vi "LDT Parse XML Status.vi"(8 "error in":errorcluster, 11 "XML Status":string="<tcsTCSStatus>\n  <tcsVersion>V1.8</tcsVersion>\n  <accessMode>Operator</accessMode>\n  <azCurrentWrap>-1</azCurrentWrap>\n  <heartbeat>2081334</heartbeat>\n  <inPositionIsTrue>true</inPositionIsTrue>\n  <m1CoverState>Closed</m1CoverState>\n  <mountGuideMode>OpenLoop</mountGuideMode>\n  <rotCurrentWrap>-1</rotCurrentWrap>\n  <tcsHealth>WARNING</tcsHealth>\n  <tcsState>ENABLED</tcsState>\n  <currentTimes>\n    <lst>\n      <hours>12</hours>\n      <minutesTime>55</minutesTime>\n      <secondsTime>41</secondsTime>\n    </lst>\n    <time>2020-09-14T20:44:15.228+00:00</time>\n  </currentTimes>\n  <limits>\n    <moonProximity>\n      <distance_deg>51.647106572866</distance_deg>\n      <proximityFlag>false</proximityFlag>\n    </moonProximity>\n    <sunProximity>\n      <distance_deg>16.531164188648</distance_deg>\n      <proximityFlag>false</proximityFlag>\n    </sunProximity>\n    <zenith>\n      <currentZD_deg>46.221286</currentZD_deg>\n      <elZenithLimit_deg>89.3</elZenithLimit_deg>\n      <inBlindSpotIsTrue>false</inBlindSpotIsTrue>\n      <timeToBlindSpot_min>-1</timeToBlindSpot_min>\n      <timeToBlindSpotExit_min>-1</timeToBlindSpotExit_min>\n    </zenith>\n    <airmass>1.4438282807451</airmass>\n    <currentTimeToObservable_min>-1</currentTimeToObservable_min>\n    <currentTimeToUnobservable_min>262</currentTimeToUnobservable_min>\n    <timeToRotLimit_min>-1</timeToRotLimit_min>\n    <timeToAzLimit_min>-1</timeToAzLimit_min>\n  </limits>\n  <pointingPositions>\n    <azElError>\n      <azError>-0.9792</azError>\n      <elError>0.1584</elError>\n    </azElError>\n    <currentAzEl>\n      <azimuth>\n        <degreesArc>194</degreesArc>\n        <minutesArc>45</minutesArc>\n        <secondsArc>0.7</secondsArc>\n      </azimuth>\n      <elevation>\n        <degreesAlt>43</degreesAlt>\n        <minutesArc>46</minutesArc>\n        <secondsArc>43.4</secondsArc>\n      </elevation>\n    </currentAzEl>\n    <currentHA>\n      <hours>0</hours>\n      <minutesTime>44</minutesTime>\n      <secondsTime>2.04</secondsTime>\n    </currentHA>\n    <currentRADec>\n      <declination>\n        <degreesDec>-10</degreesDec>\n        <minutesArc>15</minutesArc>\n        <secondsArc>25</secondsArc>\n      </declination>\n      <equinoxPrefix>J</equinoxPrefix>\n      <equinoxYear>2000</equinoxYear>\n      <frame>FK5</frame>\n      <ra>\n        <hours>12</hours>\n        <minutesTime>10</minutesTime>\n        <secondsTime>35.34</secondsTime>\n      </ra>\n    </currentRADec>\n    <currentParAngle>12.557342470137</currentParAngle>\n    <currentRotatorPositions>\n      <rotPA>342.260103</rotPA>\n      <iaa>185.2</iaa>\n      <rotIPA>0</rotIPA>\n    </currentRotatorPositions>\n    <difftrackStatus>\n      <dAz_ArcsPS>0</dAz_ArcsPS>\n      <dEl_ArcsPS>0</dEl_ArcsPS>\n      <dRA_ArcsPS>0</dRA_ArcsPS>\n      <dDec_ArcsPS>0</dDec_ArcsPS>\n    </difftrackStatus>\n    <objectPA>\n      <EqPA>-0</EqPA>\n      <AzPA>12.557342470137</AzPA>\n    </objectPA>\n    <demandAzEl>\n      <azimuth>\n        <degreesArc>194</degreesArc>\n        <minutesArc>45</minutesArc>\n        <secondsArc>3.68</secondsArc>\n      </azimuth>\n      <elevation>\n        <degreesAlt>43</degreesAlt>\n        <minutesArc>46</minutesArc>\n        <secondsArc>42.89</secondsArc>\n      </elevation>\n    </demandAzEl>\n    <demandRADec>\n      <declination>\n        <degreesDec>-10</degreesDec>\n        <minutesArc>15</minutesArc>\n        <secondsArc>25</secondsArc>\n      </declination>\n      <equinoxPrefix>J</equinoxPrefix>\n      <equinoxYear>2000</equinoxYear>\n      <frame>FK5</frame>\n      <ra>\n        <hours>12</hours>\n        <minutesTime>10</minutesTime>\n        <secondsTime>35.24</secondsTime>\n      </ra>\n    </demandRADec>\n    <demandRotatorPositions>\n      <rotPA>342.259442</rotPA>\n    </demandRotatorPositions>\n    <targetName>unspecified</targetName>\n  </pointingPositions>\n  <OffsetStatus>\n    <offsetType>SIMPLE</offsetType>\n    <userOff1>0</userOff1>\n    <userOff2>0</userOff2>\n    <handsetOff1>0</handsetOff1>\n    <handsetOff2>0</handsetOff2>\n  </OffsetStatus>\n  <axesTrackMode>All</axesTrackMode>\n  <inPositionAzIsTrue>true</inPositionAzIsTrue>\n  <inPositionElIsTrue>true</inPositionElIsTrue>\n  <inPositionRotIsTrue>true</inPositionRotIsTrue>\n  <externalTargetCfgCmdPreviewIsTrue>true</externalTargetCfgCmdPreviewIsTrue>\n</tcsTCSStatus>") -> (0 "error out":errorcluster, 3 "Telescope Status":T1)   [LabVIEW 2024, in "LDT Telescope.lvclass"]
uses:
  LDT Telescope.lvclass
  Telescope cluster Status.ctl
  typedefs/CC cluster RA and DEC.ctl
  Telescope enum Status.ctl
  Telescope.lvclass
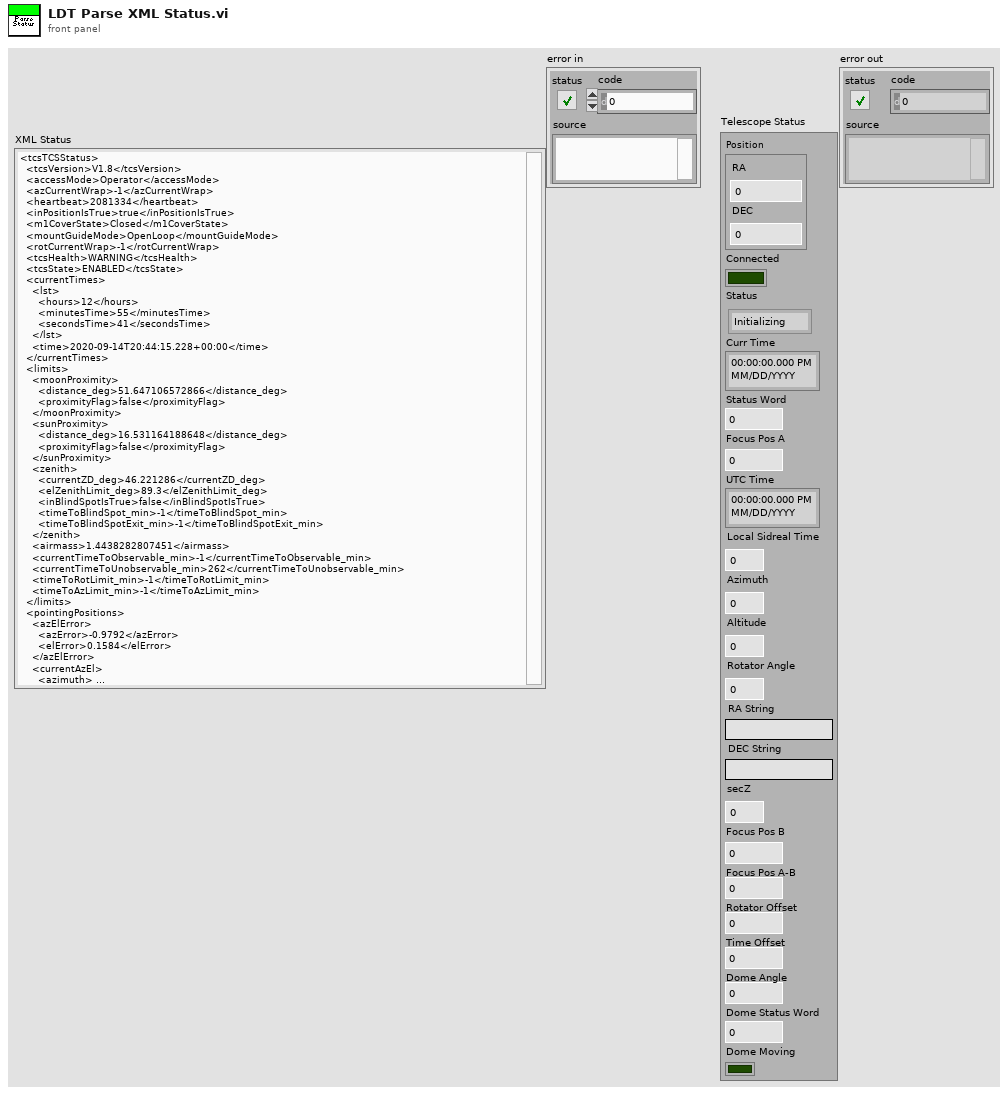
[diagram p1: front panel]
types:
  T1 = typedef "Telescope.lvclass/Telescope cluster Status.ctl" = cluster{"Position":T2, "Connected":bool, "Status":T3, "Curr Time":timestamp, "Status Word":u32, "Focus Pos A":dbl, "UTC Time":timestamp, "Local Sidreal Time":dbl, "Azimuth":dbl, "Altitude":dbl, "Rotator Angle":dbl, "RA String":string, "DEC String":string, "secZ":dbl, "Focus Pos B":dbl, "Focus Pos A-B":dbl, "Rotator Offset":dbl, "Time Offset":dbl, "Dome Angle":dbl, "Dome Status Word":u32, "Dome Moving":bool}
  T2 = typedef "CC cluster RA and DEC.ctl" = cluster{"RA":dbl, "DEC":dbl}
  T3 = typedef "Telescope.lvclass/Telescope enum Status.ctl" = enum16{"Initializing", "Ready", "Moving", "Focusing", "Error"}
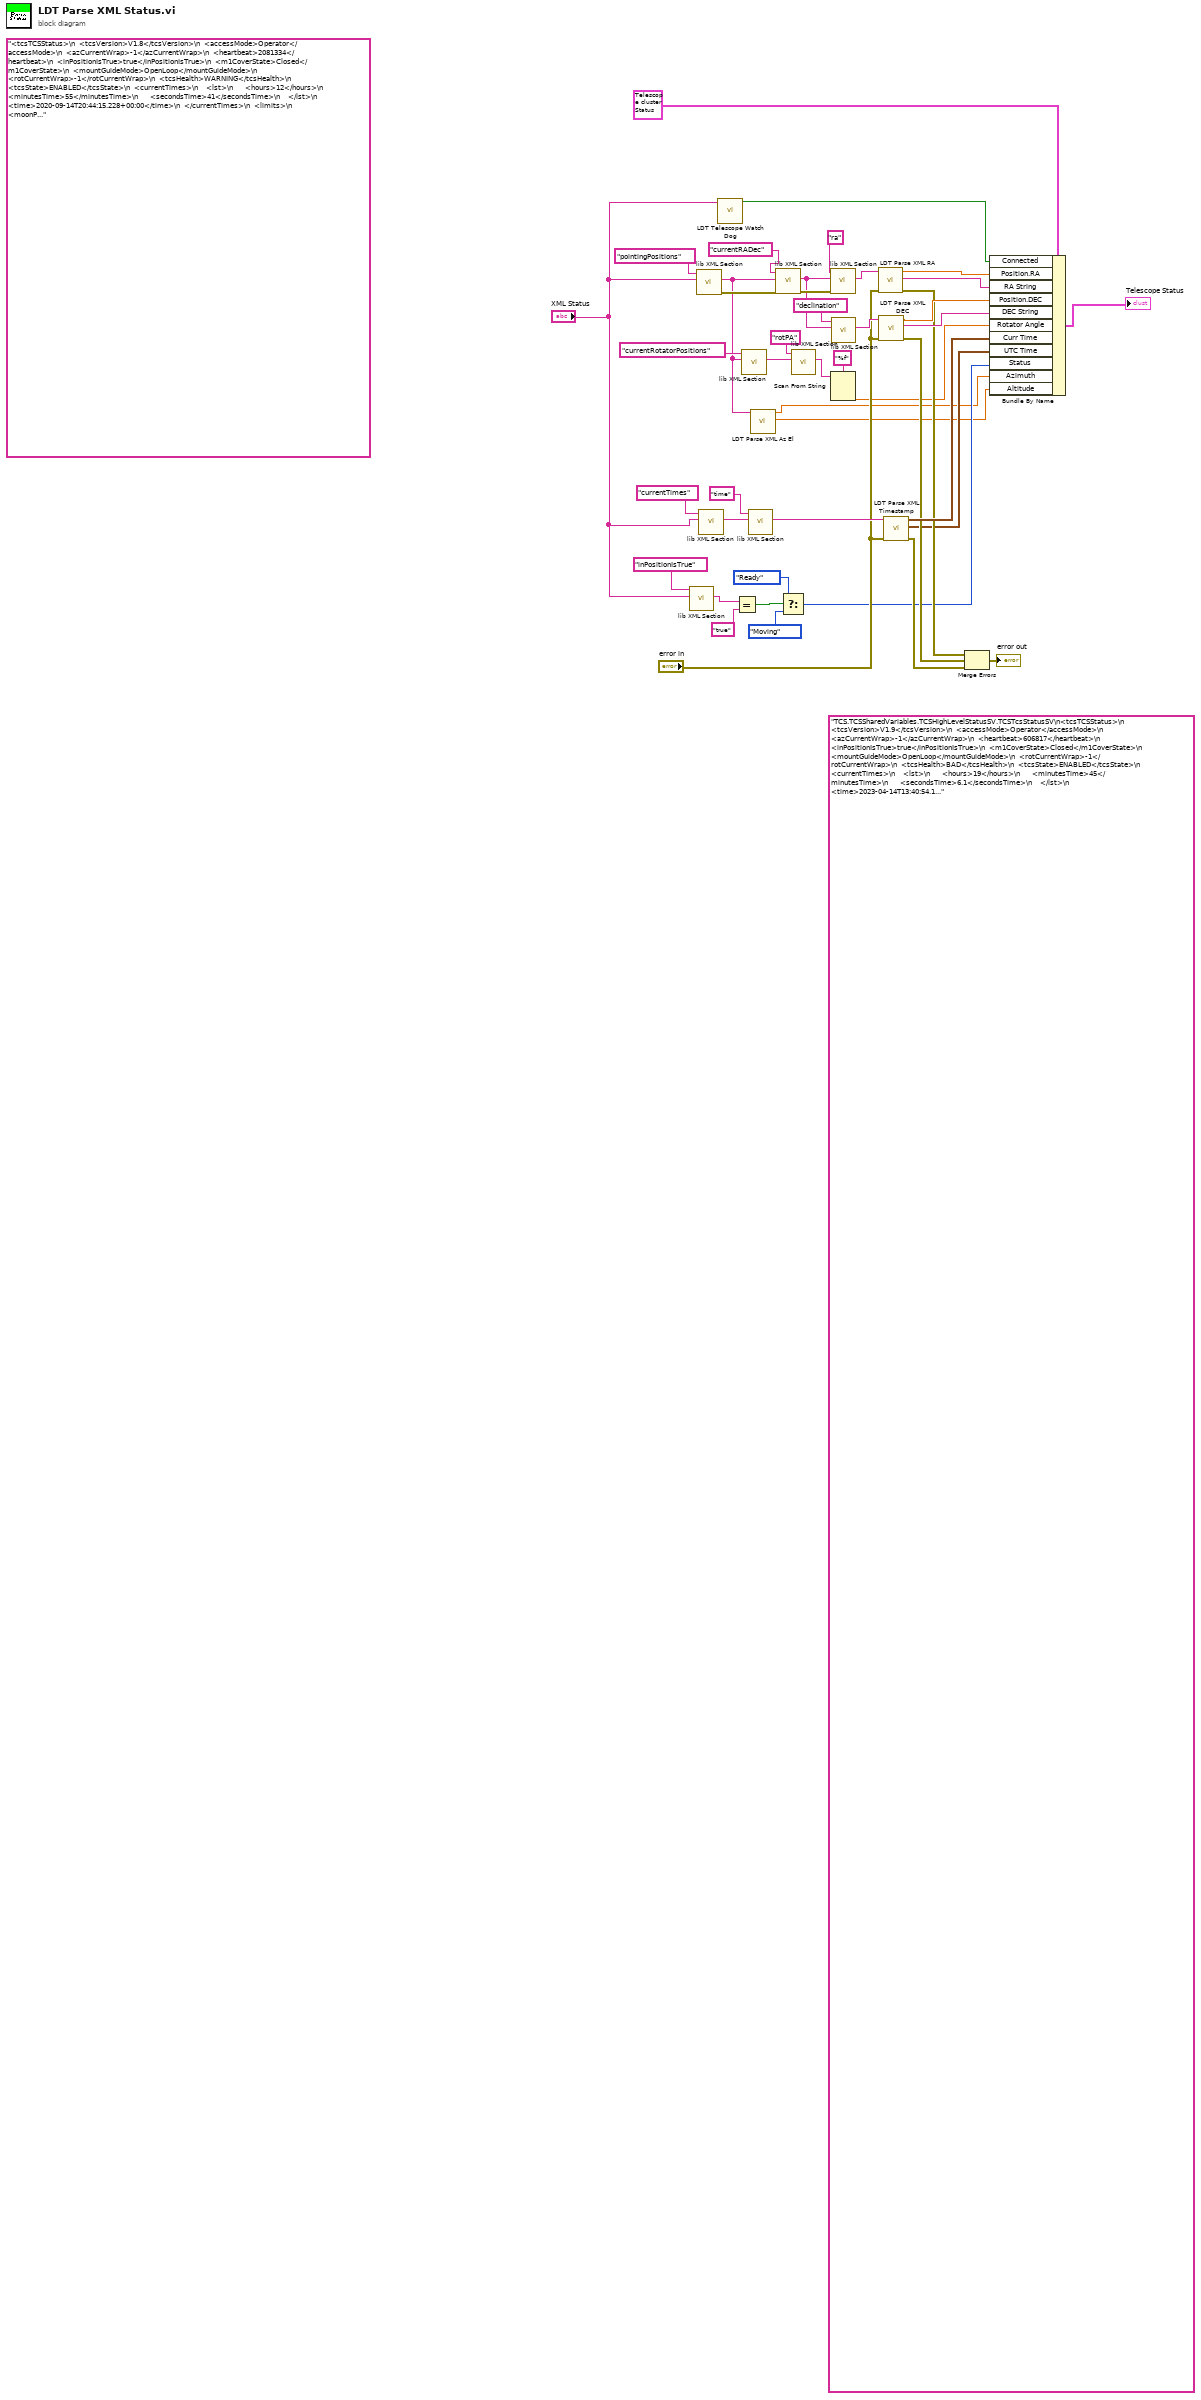
[diagram p0: block diagram]
diagram:
  (unwired) "TCS.TCSSharedVariables.TCSHighLevelStatusSV.TCSTcsStatusSV\n<tcsTCSStatus>\n  <tcsVersion>V1.9</tcsVersion>\n  <accessMode>Operator</accessMode>\n  <azCurrentWrap>-1</azCurrentWrap>\n  <heartbeat>606817</heartbeat>\n  <inPositionIsTrue>true</inPositionIsTrue>\n  <m1CoverState>Closed</m1CoverState>\n  <mountGuideMode>OpenLoop</mountGuideMode>\n  <rotCurrentWrap>-1</rotCurrentWrap>\n  <tcsHealth>BAD</tcsHealth>\n  <tcsState>ENABLED</tcsState>\n  <currentTimes>\n    <lst>\n      <hours>19</hours>\n      <minutesTime>45</minutesTime>\n      <secondsTime>6.1</secondsTime>\n    </lst>\n    <time>2023-04-14T13:40:54.171+00:00</time>\n  </currentTimes>\n  <limits>\n    <moonProximity>\n      <distance_deg>135.17188173454</distance_deg>\n      <proximityFlag>false</proximityFlag>\n    </moonProximity>\n    <sunProximity>\n      <distance_deg>85.698048093239</distance_deg>\n      <proximityFlag>false</proximityFlag>\n    </sunProximity>\n    <zenith>\n      <currentZD_deg>77.038641</currentZD_deg>\n      <elZenithLimit_deg>89.3</elZenithLimit_deg>\n      <inBlindSpotIsTrue>false</inBlindSpotIsTrue>\n      <timeToBlindSpot_min>-1</timeToBlindSpot_min>\n      <timeToBlindSpotExit_min>-1</timeToBlindSpotExit_min>\n    </zenith>\n    <airmass>4.3842110871255</airmass>\n    <currentTimeToObservable_min>-1</currentTimeToObservable_min>\n    <currentTimeToUnobservable_min>-1</currentTimeToUnobservable_min>\n    <timeToRotLimit_min>-1</timeToRotLimit_min>\n    <timeToAzLimit_min>-1</timeToAzLimit_min>\n  </limits>\n  <pointingPositions>\n    <azElError>\n      <azError>-0.288</azError>\n      <elError>0.036</elError>\n    </azElError>\n    <currentAzEl>\n      <azimuth>\n        <degreesArc>356</degreesArc>\n        <minutesArc>30</minutesArc>\n        <secondsArc>2.4</secondsArc>\n      </azimuth>\n      <elevation>\n        <degreesAlt>12</degreesAlt>\n        <minutesArc>57</minutesArc>\n        <secondsArc>40.9</secondsArc>\n      </elevation>\n    </currentAzEl>\n    <currentHA>\n      <hours>11</hours>\n      <minutesTime>26</minutesTime>\n      <secondsTime>48.74</secondsTime>\n    </currentHA>\n    <currentRADec>\n      <declination>\n        <degreesDec>68</degreesDec>\n        <minutesArc>0</minutesArc>\n        <secondsArc>0.3</secondsArc>\n      </declination>\n      <equinoxPrefix>J</equinoxPrefix>\n      <equinoxYear>2000</equinoxYear>\n      <frame>FK5</frame>\n      <ra>\n        <hours>8</hours>\n        <minutesTime>16</minutesTime>\n        <secondsTime>0.18</secondsTime>\n      </ra>\n    </currentRADec>\n    <currentParAngle>6.9879469176224</currentParAngle>\n    <currentRotatorPositions>\n      <rotPA>348.103896</rotPA>\n      <iaa>185.2</iaa>\n      <rotIPA>0</rotIPA>\n    </currentRotatorPositions>\n    <difftrackStatus>\n      <dAz_ArcsPS>0</dAz_ArcsPS>\n      <dEl_ArcsPS>0</dEl_ArcsPS>\n      <dRA_ArcsPS>0</dRA_ArcsPS>\n      <dDec_ArcsPS>0</dDec_ArcsPS>\n    </difftrackStatus>\n    <objectPA>\n      <EqPA>-0</EqPA>\n      <AzPA>6.9879469176224</AzPA>\n    </objectPA>\n    <demandAzEl>\n      <azimuth>\n        <degreesArc>356</degreesArc>\n        <minutesArc>30</minutesArc>\n        <secondsArc>3.57</secondsArc>\n      </azimuth>\n      <elevation>\n        <degreesAlt>12</degreesAlt>\n        <minutesArc>57</minutesArc>\n        <secondsArc>40.76</secondsArc>\n      </elevation>\n    </demandAzEl>\n    <demandRADec>\n      <declination>\n        <degreesDec>68</degreesDec>\n        <minutesArc>0</minutesArc>\n        <secondsArc>0.3</secondsArc>\n      </declination>\n      <equinoxPrefix>J</equinoxPrefix>\n      <equinoxYear>2000</equinoxYear>\n      <frame>FK5</frame>\n      <ra>\n        <hours>8</hours>\n        <minutesTime>16</minutesTime>\n        <secondsTime>0.03</secondsTime>\n      </ra>\n    </demandRADec>\n    <demandRotatorPositions>\n      <rotPA>348.104592</rotPA>\n    </demandRotatorPositions>\n    <targetName>MyTarget</targetName>\n  </pointingPositions>\n  <OffsetStatus>\n    <offsetType>SIMPLE</offsetType>\n    <userOff1>0</userOff1>\n    <userOff2>0</userOff2>\n    <handsetOff1>0</handsetOff1>\n    <handsetOff2>0</handsetOff2>\n  </OffsetStatus>\n  <axesTrackMode>All</axesTrackMode>\n  <inPositionAzIsTrue>true</inPositionAzIsTrue>\n  <inPositionElIsTrue>true</inPositionElIsTrue>\n  <inPositionRotIsTrue>true</inPositionRotIsTrue>\n  <externalTargetCfgCmdPreviewIsTrue>true</externalTargetCfgCmdPreviewIsTrue>\n</tcsTCSStatus>"
  (unwired) "<tcsTCSStatus>\n  <tcsVersion>V1.8</tcsVersion>\n  <accessMode>Operator</accessMode>\n  <azCurrentWrap>-1</azCurrentWrap>\n  <heartbeat>2081334</heartbeat>\n  <inPositionIsTrue>true</inPositionIsTrue>\n  <m1CoverState>Closed</m1CoverState>\n  <mountGuideMode>OpenLoop</mountGuideMode>\n  <rotCurrentWrap>-1</rotCurrentWrap>\n  <tcsHealth>WARNING</tcsHealth>\n  <tcsState>ENABLED</tcsState>\n  <currentTimes>\n    <lst>\n      <hours>12</hours>\n      <minutesTime>55</minutesTime>\n      <secondsTime>41</secondsTime>\n    </lst>\n    <time>2020-09-14T20:44:15.228+00:00</time>\n  </currentTimes>\n  <limits>\n    <moonProximity>\n      <distance_deg>51.647106572866</distance_deg>\n      <proximityFlag>false</proximityFlag>\n    </moonProximity>\n    <sunProximity>\n      <distance_deg>16.531164188648</distance_deg>\n      <proximityFlag>false</proximityFlag>\n    </sunProximity>\n    <zenith>\n      <currentZD_deg>46.221286</currentZD_deg>\n      <elZenithLimit_deg>89.3</elZenithLimit_deg>\n      <inBlindSpotIsTrue>false</inBlindSpotIsTrue>\n      <timeToBlindSpot_min>-1</timeToBlindSpot_min>\n      <timeToBlindSpotExit_min>-1</timeToBlindSpotExit_min>\n    </zenith>\n    <airmass>1.4438282807451</airmass>\n    <currentTimeToObservable_min>-1</currentTimeToObservable_min>\n    <currentTimeToUnobservable_min>262</currentTimeToUnobservable_min>\n    <timeToRotLimit_min>-1</timeToRotLimit_min>\n    <timeToAzLimit_min>-1</timeToAzLimit_min>\n  </limits>\n  <pointingPositions>\n    <azElError>\n      <azError>-0.9792</azError>\n      <elError>0.1584</elError>\n    </azElError>\n    <currentAzEl>\n      <azimuth>\n        <degreesArc>194</degreesArc>\n        <minutesArc>45</minutesArc>\n        <secondsArc>0.7</secondsArc>\n      </azimuth>\n      <elevation>\n        <degreesAlt>43</degreesAlt>\n        <minutesArc>46</minutesArc>\n        <secondsArc>43.4</secondsArc>\n      </elevation>\n    </currentAzEl>\n    <currentHA>\n      <hours>0</hours>\n      <minutesTime>44</minutesTime>\n      <secondsTime>2.04</secondsTime>\n    </currentHA>\n    <currentRADec>\n      <declination>\n        <degreesDec>-10</degreesDec>\n        <minutesArc>15</minutesArc>\n        <secondsArc>25</secondsArc>\n      </declination>\n      <equinoxPrefix>J</equinoxPrefix>\n      <equinoxYear>2000</equinoxYear>\n      <frame>FK5</frame>\n      <ra>\n        <hours>12</hours>\n        <minutesTime>10</minutesTime>\n        <secondsTime>35.34</secondsTime>\n      </ra>\n    </currentRADec>\n    <currentParAngle>12.557342470137</currentParAngle>\n    <currentRotatorPositions>\n      <rotPA>342.260103</rotPA>\n      <iaa>185.2</iaa>\n      <rotIPA>0</rotIPA>\n    </currentRotatorPositions>\n    <difftrackStatus>\n      <dAz_ArcsPS>0</dAz_ArcsPS>\n      <dEl_ArcsPS>0</dEl_ArcsPS>\n      <dRA_ArcsPS>0</dRA_ArcsPS>\n      <dDec_ArcsPS>0</dDec_ArcsPS>\n    </difftrackStatus>\n    <objectPA>\n      <EqPA>-0</EqPA>\n      <AzPA>12.557342470137</AzPA>\n    </objectPA>\n    <demandAzEl>\n      <azimuth>\n        <degreesArc>194</degreesArc>\n        <minutesArc>45</minutesArc>\n        <secondsArc>3.68</secondsArc>\n      </azimuth>\n      <elevation>\n        <degreesAlt>43</degreesAlt>\n        <minutesArc>46</minutesArc>\n        <secondsArc>42.89</secondsArc>\n      </elevation>\n    </demandAzEl>\n    <demandRADec>\n      <declination>\n        <degreesDec>-10</degreesDec>\n        <minutesArc>15</minutesArc>\n        <secondsArc>25</secondsArc>\n      </declination>\n      <equinoxPrefix>J</equinoxPrefix>\n      <equinoxYear>2000</equinoxYear>\n      <frame>FK5</frame>\n      <ra>\n        <hours>12</hours>\n        <minutesTime>10</minutesTime>\n        <secondsTime>35.24</secondsTime>\n      </ra>\n    </demandRADec>\n    <demandRotatorPositions>\n      <rotPA>342.259442</rotPA>\n    </demandRotatorPositions>\n    <targetName>unspecified</targetName>\n  </pointingPositions>\n  <OffsetStatus>\n    <offsetType>SIMPLE</offsetType>\n    <userOff1>0</userOff1>\n    <userOff2>0</userOff2>\n    <handsetOff1>0</handsetOff1>\n    <handsetOff2>0</handsetOff2>\n  </OffsetStatus>\n  <axesTrackMode>All</axesTrackMode>\n  <inPositionAzIsTrue>true</inPositionAzIsTrue>\n  <inPositionElIsTrue>true</inPositionElIsTrue>\n  <inPositionRotIsTrue>true</inPositionRotIsTrue>\n  <externalTargetCfgCmdPreviewIsTrue>true</externalTargetCfgCmdPreviewIsTrue>\n</tcsTCSStatus>"
  n1 = call "lib XML Section.vi"("XML String"="XML Status", "XML Topic"="inPositionIsTrue") -> ("XML Topic Body"=w18:string)  [unwired: 6 in, 3 out]
  n2 = call "lib XML Section.vi"("XML String"="XML Status", "XML Topic"="pointingPositions") -> ("error out"=w41:errorcluster, "XML Topic Body"=w5:string)  [unwired: 6 in, 2 out]
  n3 = call "lib XML Section.vi"("XML String"="XML Status", "XML Topic"="currentTimes") -> ("XML Topic Body"=w29:string)  [unwired: 6 in, 3 out]
  n4 = call "LDT Telescope Watch Dog.vi"("XML String"="XML Status") -> ("Connected"=w1:bool)  [unwired: 10 in]
  n5 = Equal?(x=w18, y="true") -> (x = y?=w16:bool)
  n6 = call "lib XML Section.vi"("XML String"=w5, "XML Topic"="currentRotatorPositions") -> ("XML Topic Body"=w10:string)  [unwired: 6 in, 3 out]
  n7 = call "lib XML Section.vi"("XML String"=w29, "XML Topic"="time") -> ("XML Topic Body"=w26:string)  [unwired: 6 in, 3 out]
  n8 = call "LDT Parse XML Az El.vi"("XML"=w5) -> ("Elevation"=w3:dbl, "Azimuth"=w4:dbl)  [unwired: 8 in, 1 out]
  n9 = call "lib XML Section.vi"("error in (no error)"=w41, "XML String"=w5, "XML Topic"="currentRADec") -> ("error out"=w39:errorcluster, "XML Topic Body"=w37:string)  [unwired: 5 in, 2 out]
  n10 = Select(t=Telescope_enum_Status."Ready" ("Status"), s=w16, f=Telescope_enum_Status."Moving" ("Status")) -> (s? t:f=w13:T3)
  n11 = call "lib XML Section.vi"("XML String"=w10, "XML Topic"="rotPA") -> ("XML Topic Body"=w8:string)  [unwired: 6 in, 3 out]
  n12 = call "lib XML Section.vi"("error in (no error)"=w39, "XML String"=w37, "XML Topic"="ra") -> ("XML Topic Body"=w36:string)  [unwired: 5 in, 3 out]
  n13 = Scan From String(format string="%f", input string=w8) -> (output 1=w6:dbl)  [unwired: 3 in, 3 out]
  n14 = call "lib XML Section.vi"("XML String"=w37, "XML Topic"="declination") -> ("XML Topic Body"=w35:string)  [unwired: 6 in, 3 out]
  n15 = call "LDT Parse XML RA.vi"("error in (no error)"="error in", "XML RA"=w36) -> ("error out"=w21:errorcluster, "RA string"=w33:string, "Position.RA"=w34:dbl)  [unwired: 7 in]
  n16 = call "LDT Parse XML DEC.vi"("error in (no error)"="error in", "XML Dec"=w35) -> ("error out"=w22:errorcluster, "DEC string"=w31:string, "Position.DEC"=w32:dbl)  [unwired: 7 in]
  n17 = call "LDT Parse XML Timestamp.vi"("error in"="error in", "Time"=w26) -> ("error out"=w23:errorcluster, "UTC Time"=w12:timestamp, "Local Time"=w25:timestamp)  [unwired: 7 in]
  n18 = Merge Errors(w21, w22, w23) -> (→"error out":errorcluster)
  n19 = Bundle By Name(cluster=T1 {"Position"={"RA"=0.0, "DEC"=0.0}, "Connected"=FALSE, "Status"=enum."Initializing", "Curr Time"=timestamp(0 s since 1904-01-01), "Status Word"=0, "Focus Pos A"=0.0, "UTC Time"=timestamp(0 s since 1904-01-01), "Local Sidreal Time"=0.0, "Azimuth"=0.0, "Altitude"=0.0, "Rotator Angle"=0.0, "RA String"="", "DEC String"="", "secZ"=0.0, "Focus Pos B"=0.0, "Focus Pos A-B"=0.0, "Rotator Offset"=0.0, "Time Offset"=0.0, "Dome Angle"=0.0, "Dome Status Word"=0, "Dome Moving"=FALSE} ("Telescope Status"), "Connected"=w1, "Position.RA"=w34, "RA String"=w33, "Position.DEC"=w32, "DEC String"=w31, "Rotator Angle"=w6, "Curr Time"=w25, "UTC Time"=w12, "Status"=w13, "Azimuth"=w4, "Altitude"=w3) -> (→"Telescope Status":T1)
